vi "单道符合.vi"() -> ()   [LabVIEW 2014]
panel:
  out "符合":string
  out "单道二":string
  out "单道一":string
  in  "高压":bool
  out "仪表":dbl(knob) scale=0.0..500.0
  in  "清零":bool
  in  "开始":bool
  out "状态":enum16{"初始化", "空闲", "配置", "读取", "退出"}(ring)
  out "符合":i32
  out "单道二":i32
  out "单道一":i32
  in  "道宽":u16=3000
  in  "阈值电压":u16=100
  in  "道宽":u16=3000
  in  "阈值电压":u16=100
  in  "测量时间":T1=10
  in  "符合时间3":u16
  in  "符合时间2":u16
  in  "符合时间1":u16
  in  "退出":T2
  in  "读取":bool
  in  "配置":bool
  in  "初始状态":u16(ring) items=["初始化", "空闲", "配置", "读取", "退出"]
  # "单道一"
  # "高压"
  # "单道二"
  # "符合"
  # "定标器"
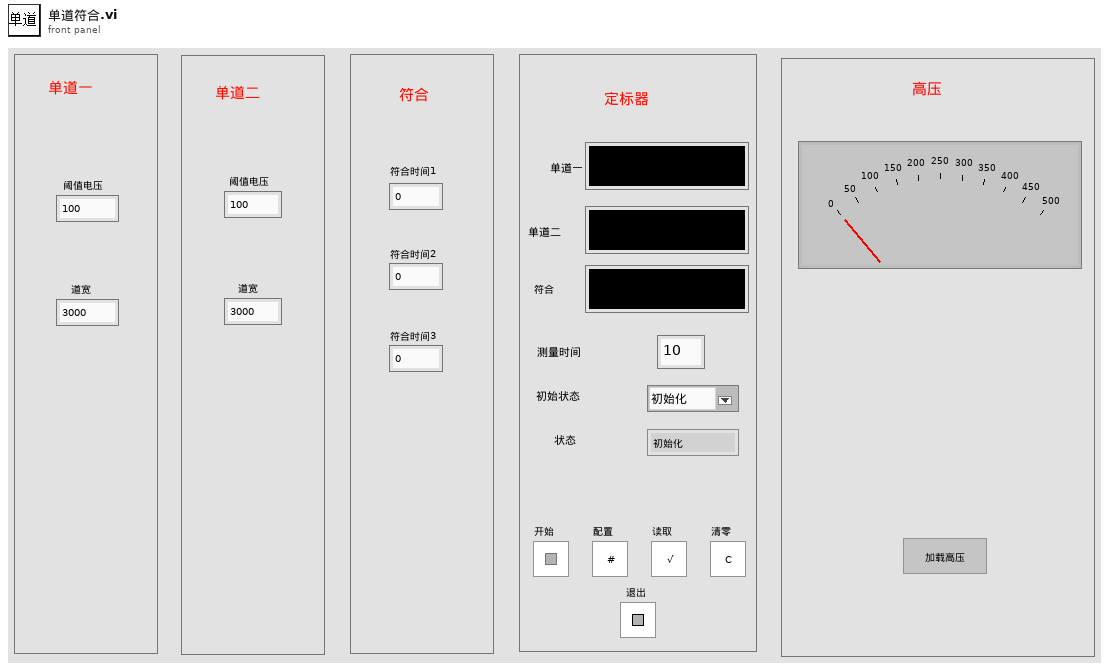
[diagram p1: front panel]
types:
  T1 = typedef "测量时间.ctl" = u16
  T2 = typedef "退出.ctl" = bool
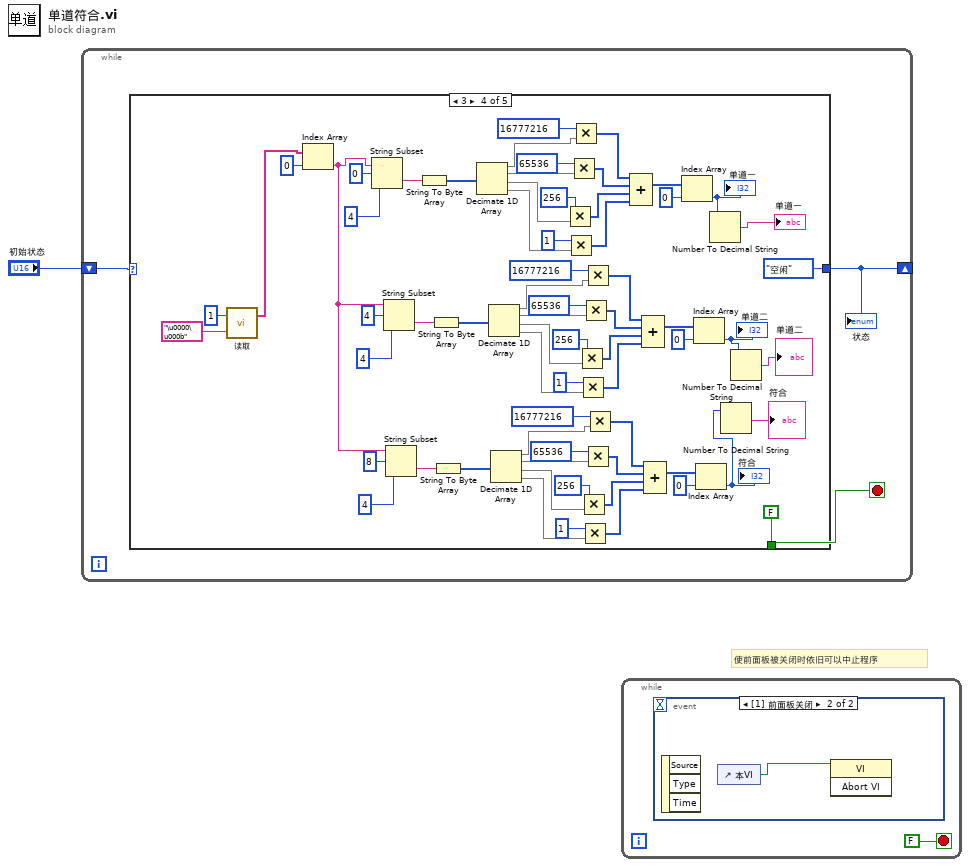
[diagram p0: block diagram]
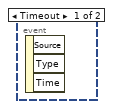
[diagram p2: hidden frame]
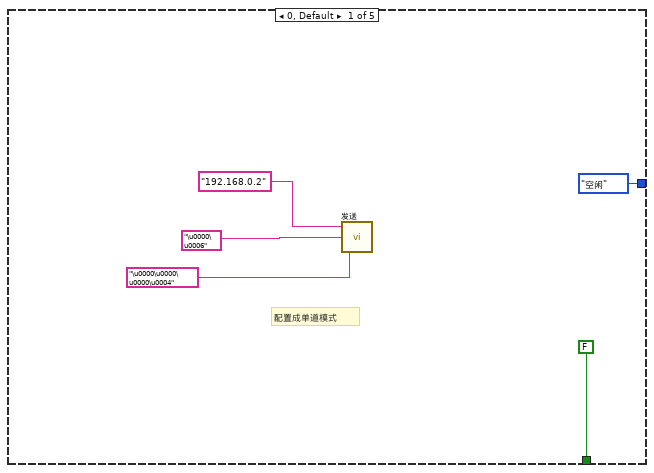
[diagram p3: hidden frame]
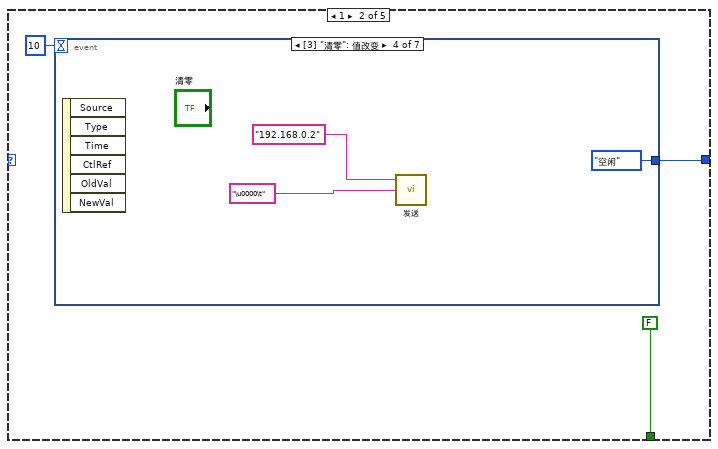
[diagram p4: hidden frame]
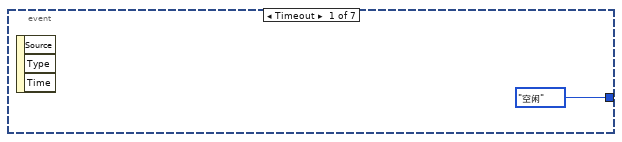
[diagram p5: hidden frame]
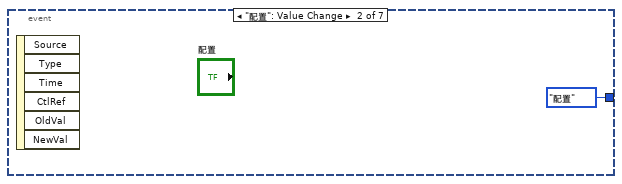
[diagram p6: hidden frame]
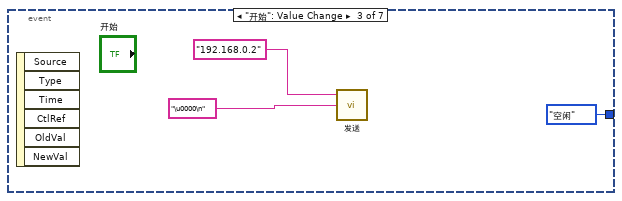
[diagram p7: hidden frame]
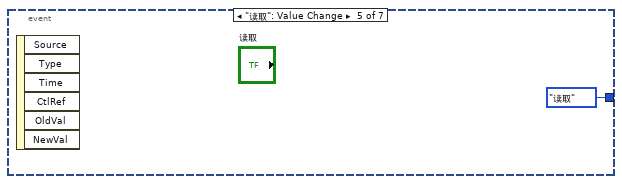
[diagram p8: hidden frame]
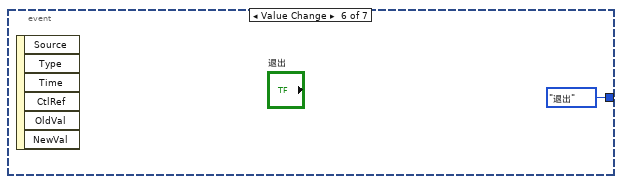
[diagram p9: hidden frame]
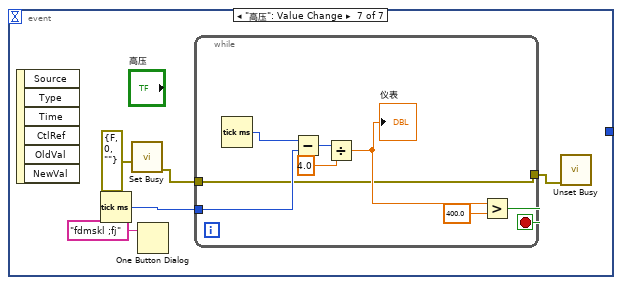
[diagram p10: hidden frame]
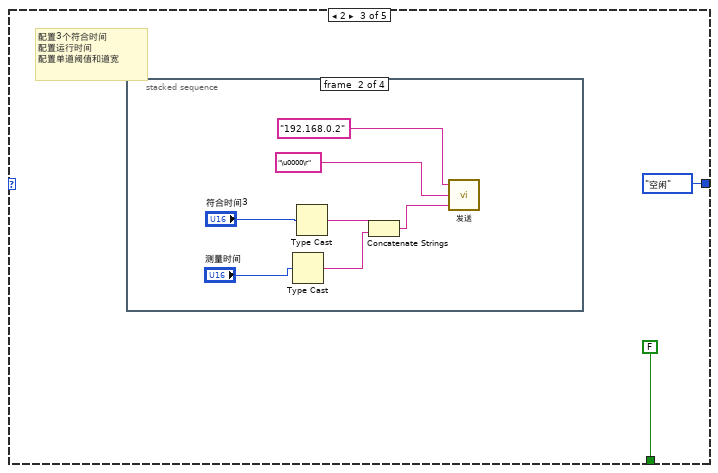
[diagram p11: hidden frame]
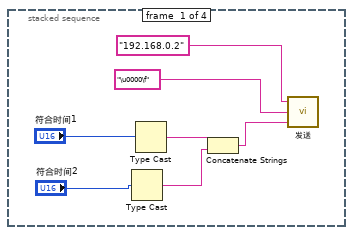
[diagram p12: hidden frame]
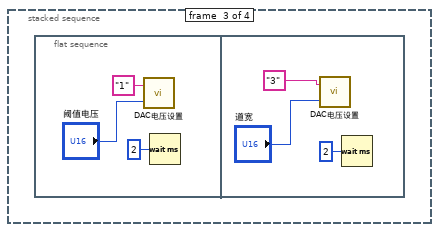
[diagram p13: hidden frame]
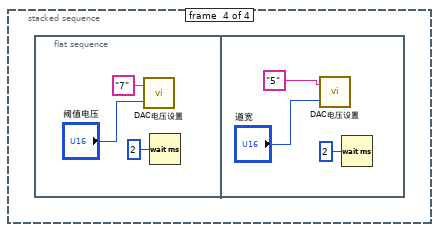
[diagram p14: hidden frame]
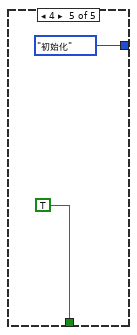
[diagram p15: hidden frame]
diagram:
  # "使前面板被关闭时依旧可以中止程序"
  n1 = while {
    shift-right: [w3] -> _
    shift-left: "初始状态" -> [w4]
    stop <- w2 stop-if-true
    n2 = case shown="3" w4 {
      tunnel: [enum16{"初始化", "空闲", "配置", "读取", "退出"}."空闲" ("初始状态") w11 enum16{"初始化", "空闲", "配置", "读取", "退出"}."空闲" ("初始状态") enum16{"初始化", "空闲", "配置", "读取", "退出"}."空闲" ("初始状态") enum16{"初始化", "空闲", "配置", "读取", "退出"}."初始化" ("初始状态")] -> w3
      tunnel: [FALSE FALSE FALSE FALSE TRUE] -> w2
      frame 0, Default {
        # "配置成单道模式"
        n3 = call "发送.vi"("数据（32bit）"="\u0000\u0000\u0000\u0004", "命令(16bit)"="\u0000\u0006", "目标IP"="192.168.0.2") -> ()  [unwired: 1 out]
      }
      frame 1 {
        n4 = event shown="[3] \"清零\": 值改变" {
          selector: _ -> [_ _ _ _ _ _ _]
          dyn-events: _ -> [_ _ _ _ _ _ _]
          timeout: 10 -> [_ _ _ _ _ _ _]
          tunnel: [enum16{"初始化", "空闲", "配置", "读取", "退出"}."空闲" ("初始状态") enum16{"初始化", "空闲", "配置", "读取", "退出"}."配置" ("初始状态") enum16{"初始化", "空闲", "配置", "读取", "退出"}."空闲" ("初始状态") enum16{"初始化", "空闲", "配置", "读取", "退出"}."空闲" ("初始状态") enum16{"初始化", "空闲", "配置", "读取", "退出"}."读取" ("初始状态") enum16{"初始化", "空闲", "配置", "读取", "退出"}."退出" ("初始状态") _] -> w11
          event Timeout {
            n5 = event-data() -> ()  [unwired: 1 in, 3 out]
          }
          event "配置": Value Change {
            n6 = event-data() -> ()  [unwired: 1 in, 6 out]
          }
          event "开始": Value Change {
            n7 = event-data() -> ()  [unwired: 1 in, 6 out]
            n8 = call "发送.vi"("命令(16bit)"="\u0000\n", "目标IP"="192.168.0.2") -> ()  [unwired: 1 in, 1 out]
          }
          event "清零": Value Change {
            n9 = event-data() -> ()  [unwired: 1 in, 6 out]
            n10 = call "发送.vi"("命令(16bit)"="\u0000\t", "目标IP"="192.168.0.2") -> ()  [unwired: 1 in, 1 out]
          }
          event "读取": Value Change {
            n11 = event-data() -> ()  [unwired: 1 in, 6 out]
          }
          event Value Change {
            n12 = event-data() -> ()  [unwired: 1 in, 6 out]
          }
          event "高压": Value Change {
            n13 = event-data() -> ()  [unwired: 1 in, 6 out]
            n14 = Tick Count (ms)() -> (millisecond timer value=w27:u32)
            n15 = call <vilib>:"Set Busy.vi"("error in (no error)"=errorcluster {"status"=FALSE, "code"=0, "source"=""}) -> ("error out"=w26:errorcluster)  [unwired: 9 in, 1 out]
            n16 = One Button Dialog(message="fdmskl ;fj" ("消息")) -> ()  [unwired: 1 in, 1 out]
            n17 = while {
              tunnel: w27 -> [w29]
              tunnel: [w28] -> w25
              tunnel: w26 -> [w28]
              stop <- w30 stop-if-true
              n18 = Tick Count (ms)() -> (millisecond timer value=w35:u32)
              n19 = Subtract(x=w35, y=w29) -> (x-y=w34:u32)
              n20 = Divide(x=w34, y=4.0) -> (x/y=w32:dbl)
              "仪表" <- w32
              n21 = Greater?(x=w32, y=400.0) -> (0:w30:bool)
            }
            n22 = call <vilib>:"Unset Busy.vi"("error in (no error)"=w25) -> ()  [unwired: 10 in, 1 out]
          }
        }
      }
      frame 2 {
        # "配置3个符合时间\n配置运行时间\n配置单道阈值和道宽"
        n23 = stacked-sequence {
          frame #0 {
            n24 = Type Cast(x="符合时间2") -> (*(type *) &x=w40:string)  [unwired: 1 in]
            n25 = Type Cast(x="符合时间1") -> (*(type *) &x=w41:string)  [unwired: 1 in]
            n26 = Concatenate Strings(w41, w40) -> (w42:string)
            n27 = call "发送.vi"("数据（32bit）"=w42, "命令(16bit)"="\u0000\f", "目标IP"="192.168.0.2") -> ()  [unwired: 1 out]
          }
          frame #1 {
            n28 = Type Cast(x="测量时间") -> (*(type *) &x=w47:string)  [unwired: 1 in]
            n29 = Type Cast(x="符合时间3") -> (*(type *) &x=w48:string)  [unwired: 1 in]
            n30 = Concatenate Strings(w48, w47) -> (w49:string)
            n31 = call "发送.vi"("数据（32bit）"=w49, "命令(16bit)"="\u0000\r", "目标IP"="192.168.0.2") -> ()  [unwired: 1 out]
          }
          frame #2 {
            n32 = flat-sequence {
              frame #0 {
                n33 = call "DAC电压设置.vi"("电压"="阈值电压", "cmd_channel(8bit)"="1") -> ()  [unwired: 1 in]
                n34 = Wait (ms)(milliseconds to wait=u32 2 ("等待时间（毫秒）")) -> ()  [unwired: 1 out]
              }
              frame #1 {
                n35 = call "DAC电压设置.vi"("电压"="道宽", "cmd_channel(8bit)"="3") -> ()  [unwired: 1 in]
                n36 = Wait (ms)(milliseconds to wait=u32 2 ("等待时间（毫秒）")) -> ()  [unwired: 1 out]
              }
            }
          }
          frame #3 {
            n37 = flat-sequence {
              frame #0 {
                n38 = call "DAC电压设置.vi"("电压"="阈值电压", "cmd_channel(8bit)"="7") -> ()  [unwired: 1 in]
                n39 = Wait (ms)(milliseconds to wait=u32 2 ("等待时间（毫秒）")) -> ()  [unwired: 1 out]
              }
              frame #1 {
                n40 = call "DAC电压设置.vi"("电压"="道宽", "cmd_channel(8bit)"="5") -> ()  [unwired: 1 in]
                n41 = Wait (ms)(milliseconds to wait=u32 2 ("等待时间（毫秒）")) -> ()  [unwired: 1 out]
              }
            }
          }
        }
      }
      frame 3 {
        n42 = call "读取.vi"("命令"="\u0000\u000b", "帧数"=1) -> ("数组"=w109:string[])  [unwired: 1 out]
        n43 = Index Array(array=w109, index=0 ("索引")) -> (element=w70:string)
        n44 = String Subset(string=w70, offset (0)=0 ("偏移量(0)"), length (rest)=4 ("长度（剩余）")) -> (substring=w113:string)
        n45 = String Subset(string=w70, offset (0)=4 ("偏移量(0)"), length (rest)=4 ("长度（剩余）")) -> (substring=w94:string)
        n46 = String Subset(string=w70, offset (0)=8 ("偏移量(0)"), length (rest)=4 ("长度（剩余）")) -> (substring=w74:string)
        n47 = String To Byte Array(string=w113) -> (unsigned byte array=w112:u8[])
        n48 = String To Byte Array(string=w94) -> (unsigned byte array=w93:u8[])
        n49 = String To Byte Array(string=w74) -> (unsigned byte array=w73:u8[])
        n50 = Decimate 1D Array(w112) -> (w114:u8[], w115:u8[], w125:u8[], w124:u8[])
        n51 = Decimate 1D Array(w93) -> (w95:u8[], w96:u8[], w106:u8[], w105:u8[])
        n52 = Decimate 1D Array(w73) -> (w75:u8[], w76:u8[], w86:u8[], w85:u8[])
        n53 = Multiply(x=256, y=w125) -> (x*y=w120:i32[])
        n54 = Multiply(x=1, y=w124) -> (x*y=w121:i32[])
        n55 = Multiply(x=65536, y=w115) -> (x*y=w117:i32[])
        n56 = Multiply(x=16777216, y=w114) -> (x*y=w116:i32[])
        n57 = Multiply(x=256, y=w106) -> (x*y=w101:i32[])
        n58 = Multiply(x=1, y=w105) -> (x*y=w102:i32[])
        n59 = Multiply(x=256, y=w86) -> (x*y=w81:i32[])
        n60 = Multiply(x=1, y=w85) -> (x*y=w82:i32[])
        n61 = Multiply(x=65536, y=w96) -> (x*y=w98:i32[])
        n62 = Multiply(x=16777216, y=w95) -> (x*y=w97:i32[])
        n63 = Multiply(x=65536, y=w76) -> (x*y=w78:i32[])
        n64 = Multiply(x=16777216, y=w75) -> (x*y=w77:i32[])
        n65 = Compound Arithmetic op=ADD(w116, w117, w120, w121) -> (w111:i32[])
        n66 = Compound Arithmetic op=ADD(w97, w98, w101, w102) -> (w92:i32[])
        n67 = Compound Arithmetic op=ADD(w77, w78, w81, w82) -> (w72:i32[])
        n68 = Index Array(array=w111, index=0 ("索引")) -> (element=w68:i32)
        "单道一" <- w68
        n69 = Index Array(array=w92, index=0 ("索引")) -> (element=w64:i32)
        "单道二" <- w64
        n70 = Index Array(array=w72, index=0 ("索引")) -> (element=w66:i32)
        "符合" <- w66
        n71 = Number To Decimal String(number=w68) -> (decimal integer string=→"单道一":string)  [unwired: 1 in]
        n72 = Number To Decimal String(number=w66) -> (decimal integer string=→"符合":string)  [unwired: 1 in]
        n73 = Number To Decimal String(number=w64) -> (decimal integer string=→"单道二":string)  [unwired: 1 in]
      }
      frame 4 {
      }
    }
    "状态" <- w3
  }
  n74 = while {
    stop <- FALSE stop-if-true
    n75 = event shown="[1] 前面板关闭" {
      selector: _ -> [_ _]
      dyn-events: _ -> [_ _]
      timeout: _ -> [_ _]
      event Timeout {
        n76 = event-data() -> ()  [unwired: 1 in, 3 out]
      }
      event Panel Close {
        n77 = event-data() -> ()  [unwired: 1 in, 3 out]
        n78 = control-ref of="本VI"() -> (w134:refnum<vi>)
        n79 = invoke class="VI" method="Abort VI"(reference=w134) -> ()  [unwired: 2 in, 3 out]
      }
    }
  }
